vi "Move.vi"(8 "error in (no error)":errorcluster, 9 "New path":string, 10 "Path":string, 11 "WebDAV in":refnum<class "WebDAV.lvclass">) -> (0 "error out":errorcluster, 3 "WebDAV out":refnum<class "WebDAV.lvclass">)   [LabVIEW 2015, in "RT Management.lvlib" / "WebDAV.lvclass"]
uses:
  WebDAV.lvclass
  WebDAV.lvclass/WebDAV.ctl
  Get Session.vi
  File Transfer Behavior/File Transfer Behavior.lvclass
  <vilib>/WebDAVClient/NI_WebDAV.lvlib
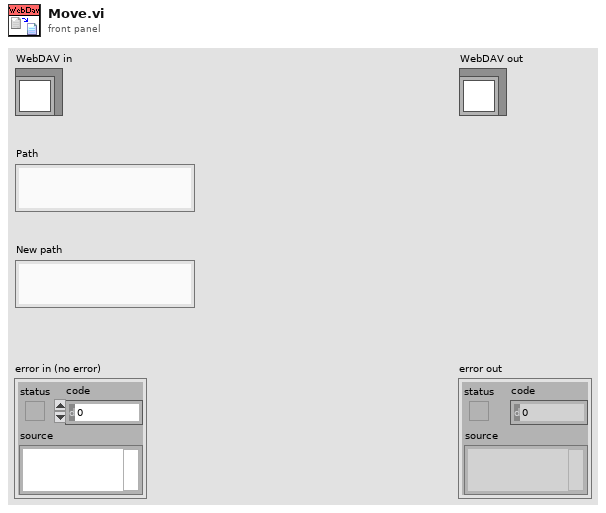
[diagram p1: front panel]
types:
  T1 = typedef "NI_WebDAV.lvlib/SessionHandle.ctl" = refnum<k1>
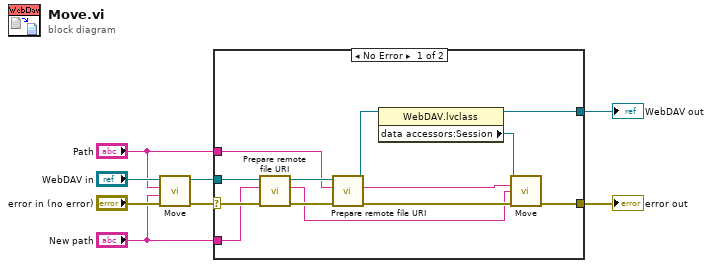
[diagram p0: block diagram]
diagram:
  n1 = call-parent <vilib>:"Move.vi"("error in (no error)"="error in (no error)", "New path"="New path", "Path"="Path", "File Transfer Behavior in"="WebDAV in") -> ("error out"=w5:errorcluster, "File Transfer Behavior out"=w3:refnum<class "WebDAV.lvclass">)  [unwired: 6 in]
  n2 = case shown="No Error" w5 {
    selector: w5 -> [w17 w23]
    tunnel: [w20 w23] -> w8
    tunnel: w3 -> [w16 w22]
    tunnel: [w18 w22] -> w7
    tunnel: "New path" -> [w12 _]
    tunnel: "Path" -> [w11 _]
    frame No Error {
      n3 = call "Prepare remote file URI.vi"("error in (no error)"=w17, "Remote path"=w12, "WebDAV in"=w16) -> ("error out"=w15:errorcluster, "Remote file URI"=w9:string, "WebDAV out"=w14:refnum<class "WebDAV.lvclass">)  [unwired: 6 in]
      n4 = call "Prepare remote file URI.vi"("error in (no error)"=w15, "Remote path"=w11, "WebDAV in"=w14) -> ("error out"=w21:errorcluster, "Remote file URI"=w10:string, "WebDAV out"=w13:refnum<class "WebDAV.lvclass">)  [unwired: 6 in]
      n5 = property class="WebDAV.lvclass"(reference=w13) -> (reference out=w18:refnum<class "WebDAV.lvclass">, "data accessors:Session"=w19:T1)  [unwired: 1 in, 1 out]
      n6 = call <vilib>:"Move.vi"("session handle"=w19, "relative source uri"=w10, "relative destination uri"=w9, "error in (no error)"=w21) -> ("error out"=w20:errorcluster)  [unwired: 10 in, 1 out]
    }
    frame Error {
    }
  }
  "error out" <- w8
  "WebDAV out" <- w7
